vi "main.vi"() -> ()   [LabVIEW 2018]
uses:
  C:/Program Files (x86)/National Instruments/LabVIEW 2018/vi.lib/ActorFramework/Actor/Actor.lvclass
  <vilib>/ActorFramework/Message Enqueuer/Message Enqueuer.lvclass/Message Enqueuer.ctl
  <vilib>/Utility/miscctls.llb/LVPoint32TypeDef.ctl
  <vilib>/ActorFramework/Message Enqueuer/Enqueue.vi
  C:/Program Files (x86)/National Instruments/LabVIEW 2018/vi.lib/ActorFramework/Message/Message.lvclass
  <vilib>/ActorFramework/Stop Msg/Stop Msg.lvclass
  <vilib>/ActorFramework/Message Priority Queue/Priority Enqueue.vi
  <vilib>/Utility/cursorutil.llb/Set Cursor (Icon Pict).vi
  <vilib>/ActorFramework/Actor/Actor.lvclass
panel:
  out "编译执行状态":string caption="文本程序"
  in  "工具-执行":bool
  in  "工具-编译":bool
  in  "工具-导出py":bool
  in  "工具-另存为":bool
  in  "工具-保存":bool
  in  "工具-新建":bool
  in  "工具-打开":bool
  in  "工具-下载":bool
  out "保存状态":string
  out "文本程序":string
  in  "图形程序":picture[][](array[picture])
  out "备注":string[][](array[string])
  in  "辅助线":picture
  in  "连接线":picture
  in  "交互信息":string[][](array[string])
  in  "编辑控件类型":bool
  out "编辑控件":bool
  in  "全部控件":T1(array[cluster])
  in  "控件类型":cluster{"二维图片":picture, "类型名称":string}[](array[cluster])
  in  "控件列表":T2(array[cluster])
  in  "工具-帮助":bool
  in  "关键字":string[][](array[string])
  in  "执行语句":string[][](array[string])
  in  "图片名称":string[][](array[string])
  in  "停止":bool
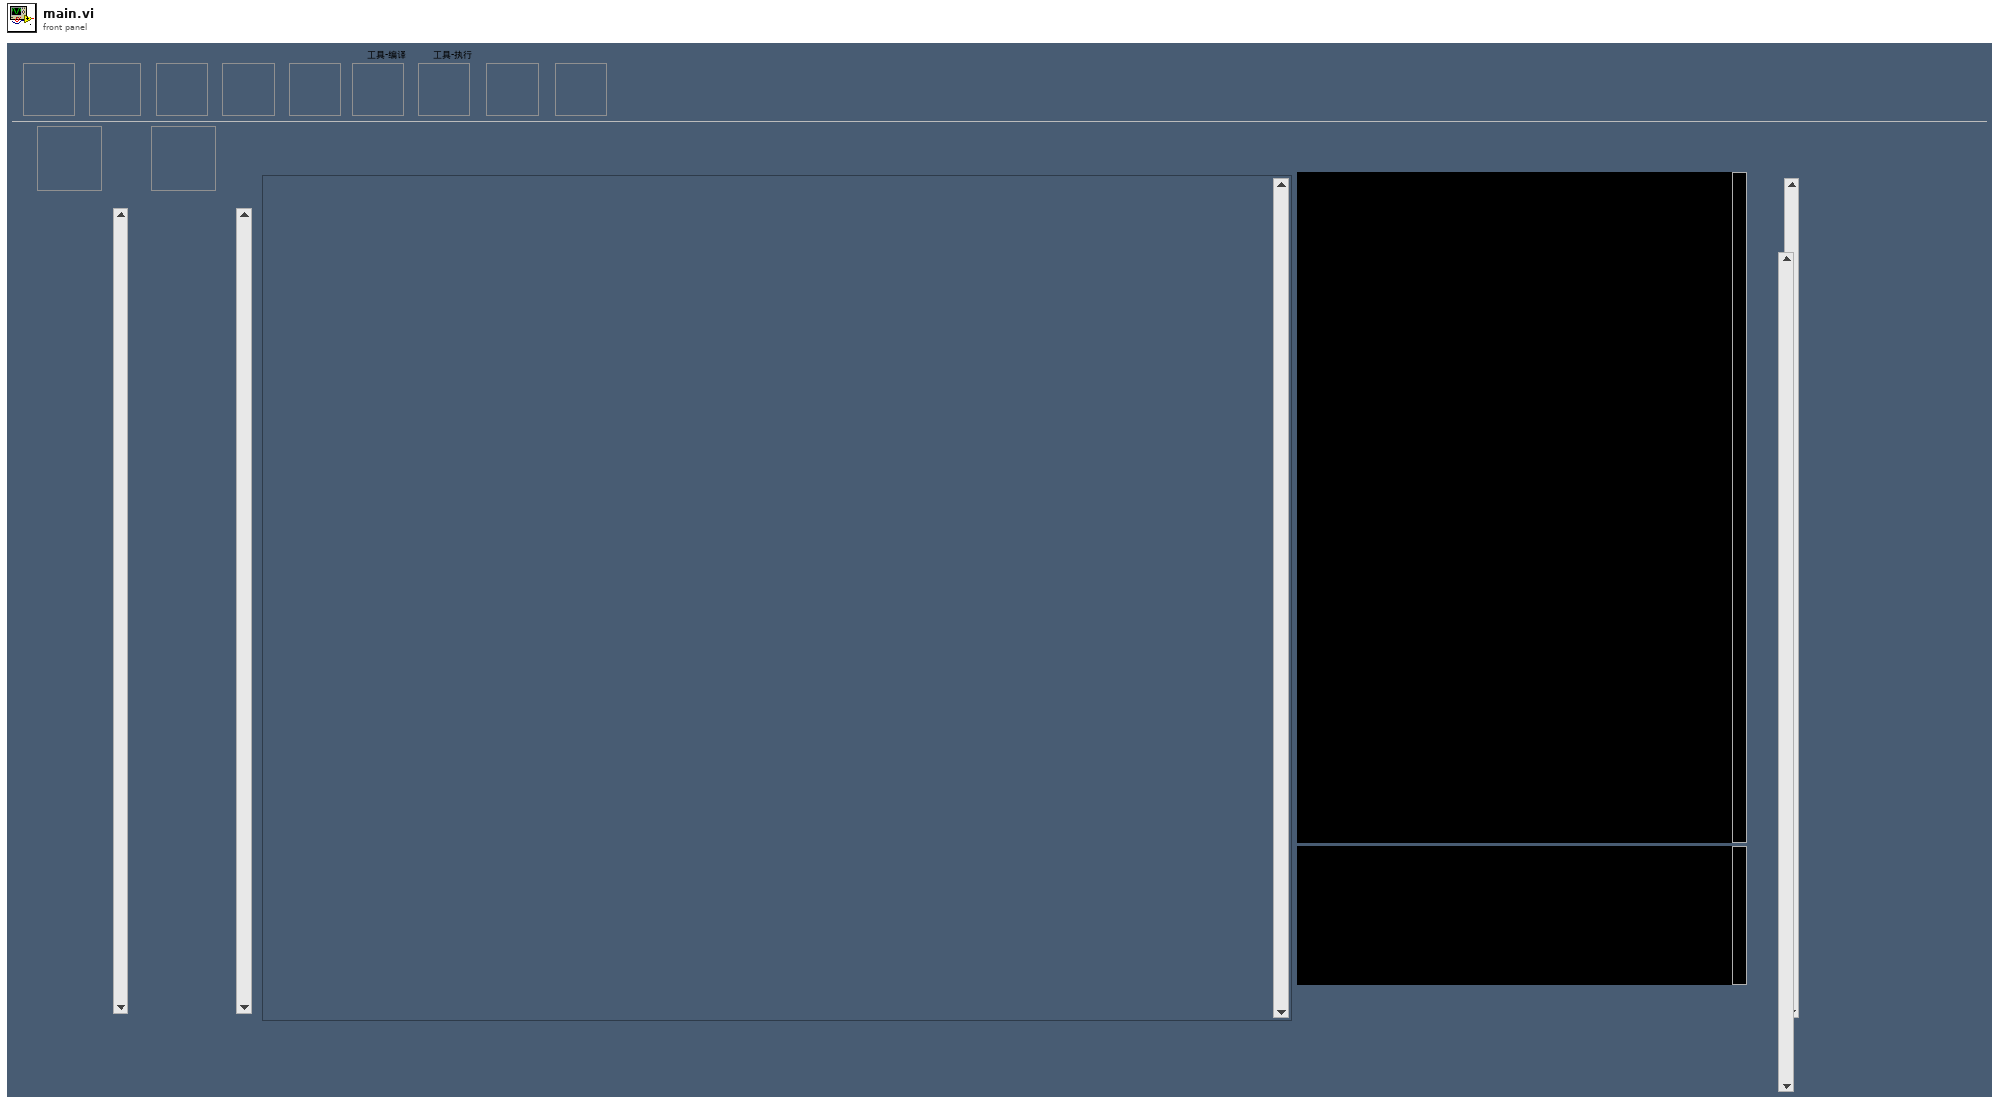
[diagram p1: front panel]
types:
  T1 = cluster{"图片":picture, "名称":string, "文本程序":string, "关键字":string}[][]
  T2 = cluster{"图片":picture, "名称":string, "文本程序":string, "关键字":string}[]
  T3 = cluster{"图形程序":refnum<vi>, "辅助线":refnum<vi>, "图片名称":refnum<vi>, "执行语句":refnum<vi>, "文本程序":refnum<vi>, "控件类型":refnum<vi>, "控件列表":refnum<vi>, "全部控件":refnum<vi>, "关键字":refnum<vi>, "连接线":refnum<vi>, "交互信息":refnum<vi>, "备注":refnum<vi>, "保存状态":refnum<vi>, "VI引用句柄":refnum<vi>, "编译执行状态":refnum<vi>}
  T4 = typedef "LVPoint32TypeDef.ctl" = cluster{"Horizontal":i32, "Vertical":i32}
  T5 = typedef "LVRectTypeDef.ctl" = cluster{"Left":i16, "Top":i16, "Right":i16, "Bottom":i16}
  T6 = typedef "LVPositionTypeDef.ctl" = cluster{"Left":i32, "Top":i32}
  T7 = typedef "eventvkey.ctl" = enum16{"ASCII", "Enter", "Return", "Shift", "Ctrl", "Alt", "Cmd", "Opt", "Caps", "NumLock", "Clear", "Break", "Up", "Down", "Left", "Right", "Insert", "Delete", "Home", "End", "PageUp", "PageDown", "Escape", "Help", "Pause", "ScrollLock", "F1", "F2", "F3", "F4", "F5", "F6", "F7", "F8", "F9", "F10", "F11", "F12", "F13", "F14", "F15", "F16", "F17", "F18", "F19", "F20", "F21", "F22", "F23", "F24", "Play", "VolumeUp", "VolumeDown", "Mute", "Two Byte Char"}
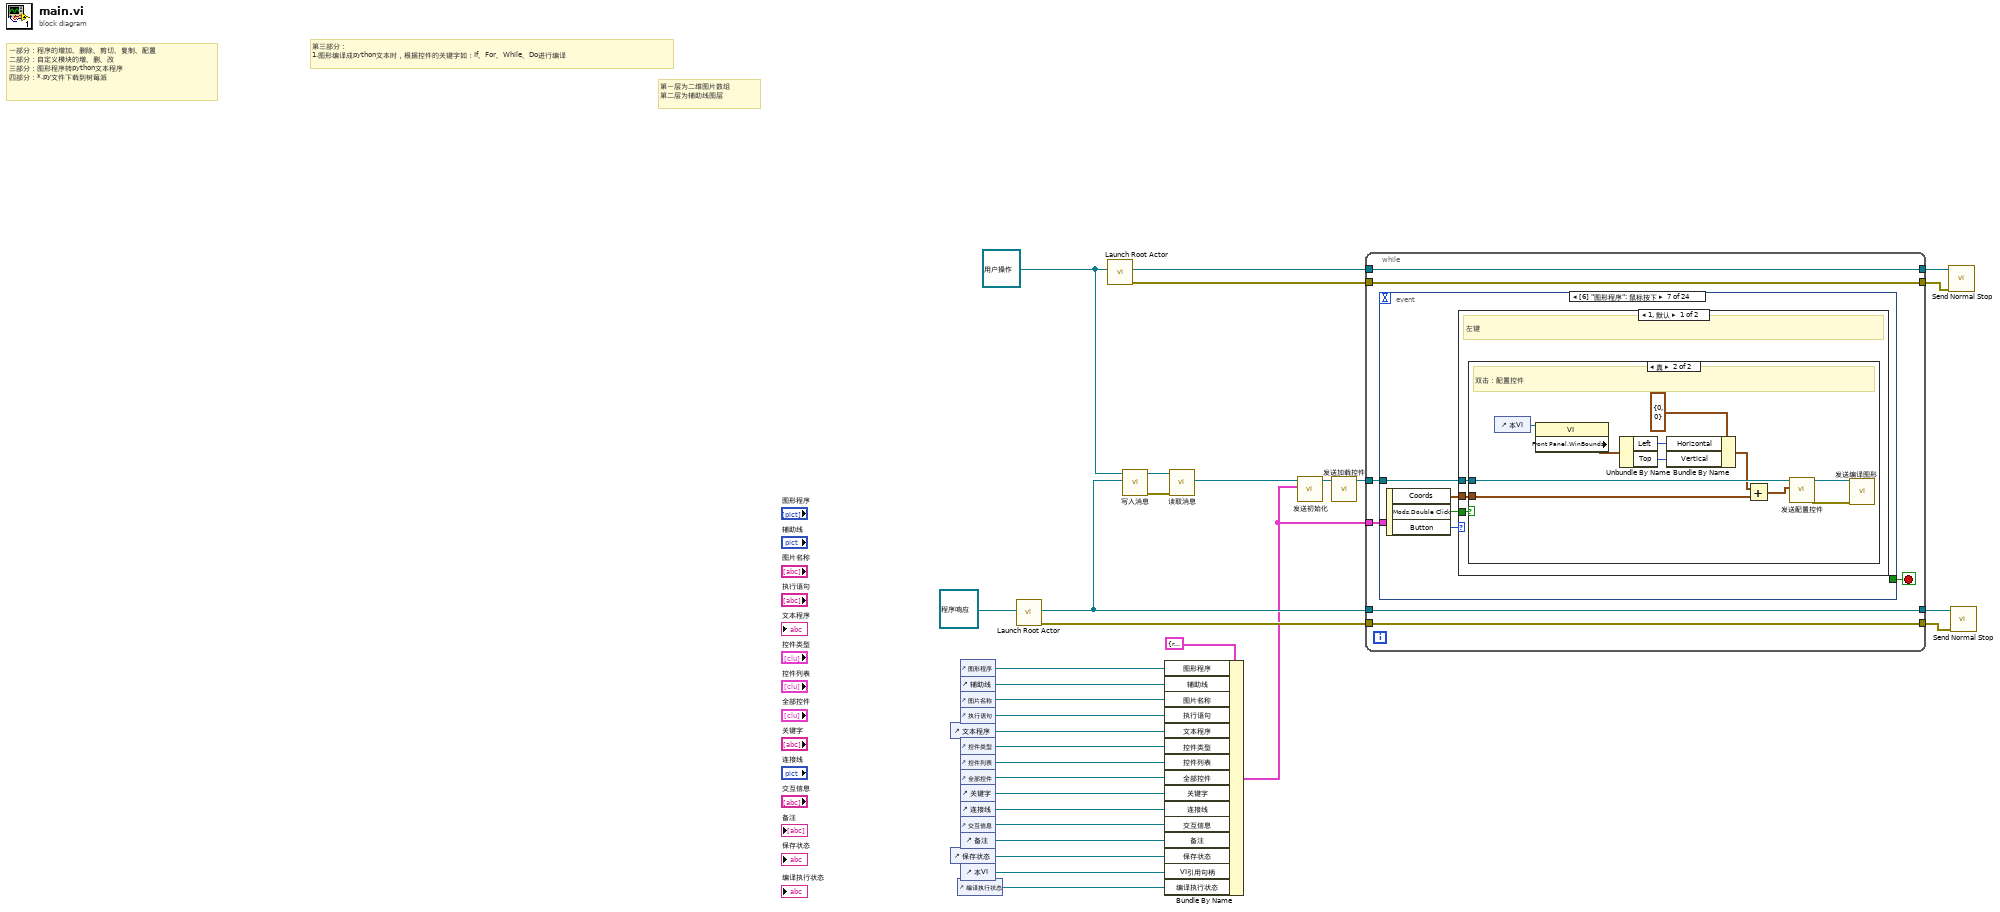
[diagram p0: block diagram]
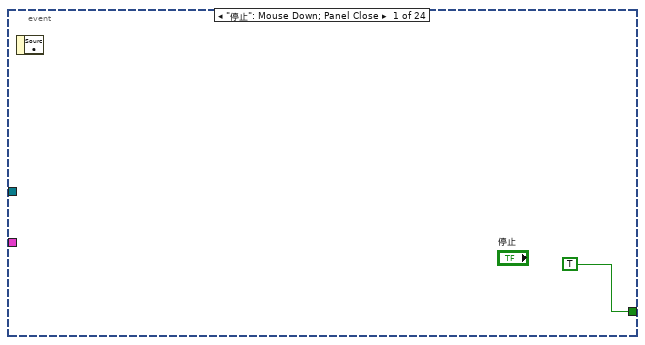
[diagram p2: hidden frame]
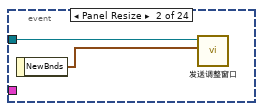
[diagram p3: hidden frame]
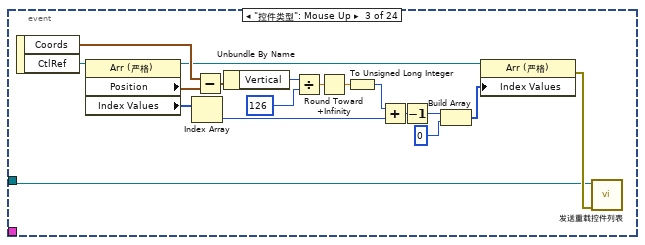
[diagram p4: hidden frame]
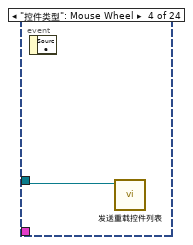
[diagram p5: hidden frame]
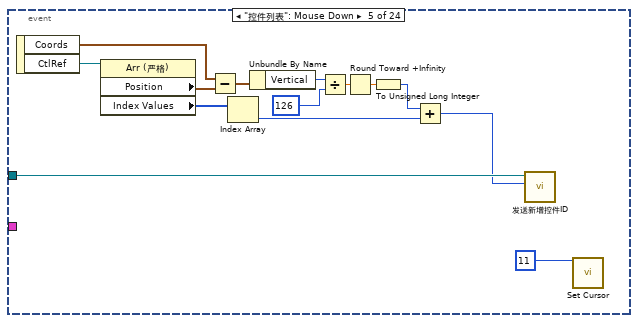
[diagram p6: hidden frame]
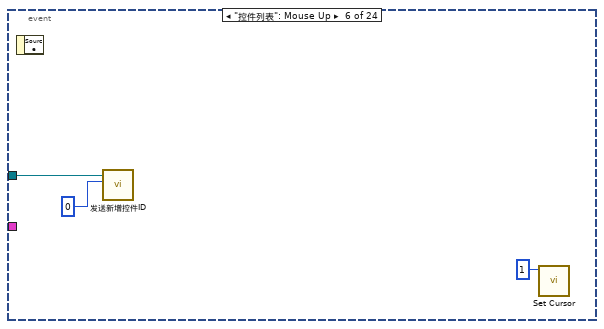
[diagram p7: hidden frame]
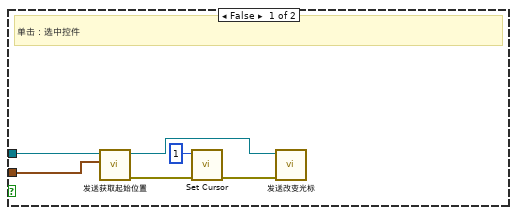
[diagram p8: hidden frame]
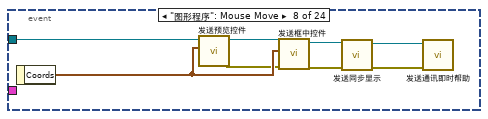
[diagram p10: hidden frame]
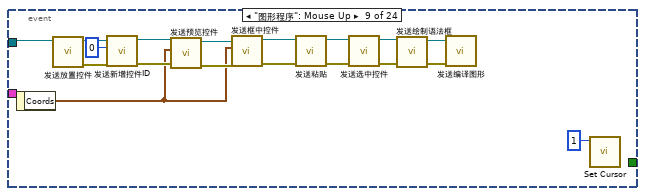
[diagram p11: hidden frame]
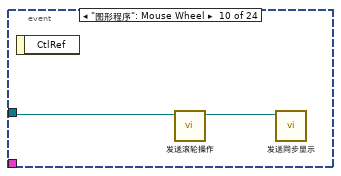
[diagram p12: hidden frame]
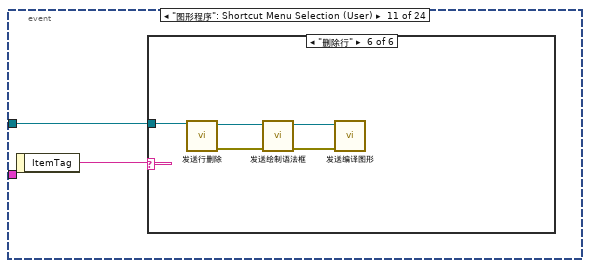
[diagram p13: hidden frame]
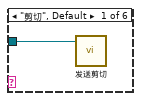
[diagram p14: hidden frame]
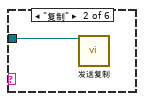
[diagram p15: hidden frame]
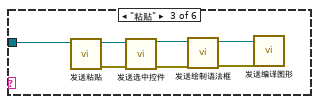
[diagram p16: hidden frame]
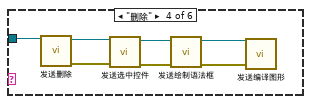
[diagram p17: hidden frame]
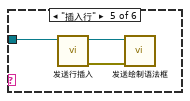
[diagram p18: hidden frame]
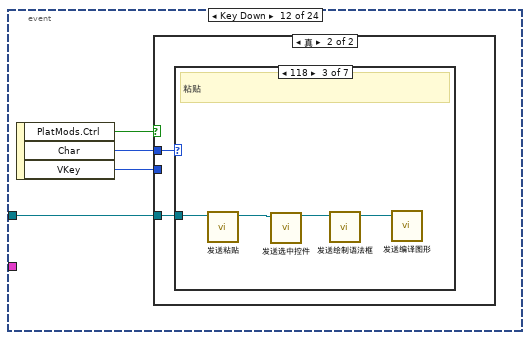
[diagram p19: hidden frame]
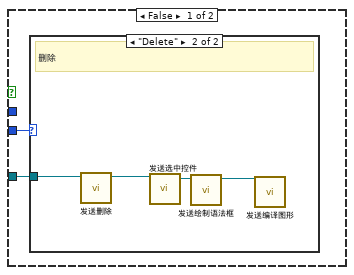
[diagram p20: hidden frame]
diagram:
  w29 = refnum<class "用户操作.lvclass"> refnum ("用户操作.lvlib:用户操作.lvclass")
  # "第三部分：\n1.图形编译成python文本时，根据控件的关键字如：If、For、While、Do进行编译"
  # "一部分：程序的增加、删除、剪切、复制、配置\n二部分：自定义模块的增、删、改\n三部分：图形程序转python文本程序\n四部分：*.py文件下载到树莓派"
  # "第一层为二维图片数组\n第二层为辅助线图层"
  n1 = control-ref of="文本程序"() -> (w16:refnum<vi>)
  n2 = control-ref of="保存状态"() -> (w7:refnum<vi>)
  n3 = control-ref of="编译执行状态"() -> (w2:refnum<vi>)
  n4 = control-ref of="图形程序"() -> (w20:refnum<vi>)
  n5 = control-ref of="辅助线"() -> (w19:refnum<vi>)
  n6 = control-ref of="图片名称"() -> (w18:refnum<vi>)
  n7 = control-ref of="执行语句"() -> (w17:refnum<vi>)
  n8 = control-ref of="控件类型"() -> (w11:refnum<vi>)
  n9 = control-ref of="控件列表"() -> (w12:refnum<vi>)
  n10 = control-ref of="全部控件"() -> (w10:refnum<vi>)
  n11 = control-ref of="关键字"() -> (w15:refnum<vi>)
  n12 = control-ref of="连接线"() -> (w14:refnum<vi>)
  n13 = control-ref of="交互信息"() -> (w9:refnum<vi>)
  n14 = control-ref of="备注"() -> (w8:refnum<vi>)
  n15 = control-ref of="本VI"() -> (w5:refnum<vi>)
  n16 = call <vilib>:"Launch Root Actor.vi"("Actor"=refnum<class "程序响应.lvclass"> refnum ("程序响应.lvlib:程序响应.lvclass")) -> ("error out"=w24:errorcluster, "Actor's Enqueuer"=w28:refnum<class "Message Enqueuer.lvclass">)  [unwired: 9 in]
  n17 = call <vilib>:"Launch Root Actor.vi"("Actor"=w29) -> ("error out"=w22:errorcluster, "Actor's Enqueuer"=w27:refnum<class "Message Enqueuer.lvclass">)  [unwired: 9 in]
  n18 = call-dynamic "写入消息.vi"("操作者框架:消息待入队列"=w28, "用户操作输入"=w29) -> ("error out"=w30:errorcluster, "用户操作输出"=w31:refnum<class "用户操作.lvclass">)  [unwired: 8 in]
  n19 = Bundle By Name(cluster=T3 {"图形程序"=refnum, "辅助线"=refnum, "图片名称"=refnum, "执行语句"=refnum, "文本程序"=refnum, "控件类型"=refnum, "控件列表"=refnum, "全部控件"=refnum, "关键字"=refnum, "连接线"=refnum, "交互信息"=refnum, "备注"=refnum, "保存状态"=refnum, "VI引用句柄"=refnum, "编译执行状态"=refnum} ("初始数据"), "图形程序"=w20, "辅助线"=w19, "图片名称"=w18, "执行语句"=w17, "文本程序"=w16, "控件类型"=w11, "控件列表"=w12, "全部控件"=w10, "关键字"=w15, "连接线"=w14, "交互信息"=w9, "备注"=w8, "保存状态"=w7, "VI引用句柄"=w5, "编译执行状态"=w2) -> (w1:T3)
  n20 = call-dynamic "读取消息.vi"("error in (no error)"=w30, "用户操作输入"=w31) -> ("操作者框架:消息待入队列"=w4:refnum<class "Message Enqueuer.lvclass">)  [unwired: 7 in, 2 out]
  n21 = call "发送初始化.vi"("初始数据"=w1, "Message Enqueuer"=w4) -> ("Message Enqueuer out"=w3:refnum<class "Message Enqueuer.lvclass">)  [unwired: 8 in, 1 out]
  n22 = call "发送加载控件.vi"("Message Enqueuer"=w3) -> ("Message Enqueuer out"=w13:refnum<class "Message Enqueuer.lvclass">)  [unwired: 9 in, 1 out]
  n23 = while {
    tunnel: w28 -> [w37]
    tunnel: w13 -> [w39]
    tunnel: w27 -> [w38]
    tunnel: [w38] -> w26
    tunnel: [w37] -> w25
    tunnel: w24 -> [w36]
    tunnel: [w36] -> w23
    tunnel: w22 -> [w35]
    tunnel: [w35] -> w21
    tunnel: w1 -> [w33]
    stop <- w34 stop-if-true
    n24 = event shown="[6] \"图形程序\": 鼠标按下" {
      selector: _ -> [_ _ _ _ _ _ _ _ _ _ _ _ _ _ _ _ _ _ _ _ _ _ _ _]
      dyn-events: _ -> [_ _ _ _ _ _ _ _ _ _ _ _ _ _ _ _ _ _ _ _ _ _ _ _]
      timeout: _ -> [_ _ _ _ _ _ _ _ _ _ _ _ _ _ _ _ _ _ _ _ _ _ _ _]
      tunnel: w39 -> [_ w42 w43 w61 w66 w78 w82 w110 w125 w129 w131 w157 w183 w186 w188 w193 w194 w195 w197 w198 w199 w201 w202 w204]
      tunnel: [TRUE _ _ _ _ _ _ _ _ _ _ _ _ _ _ _ _ _ _ _ _ _ _ _] -> w34
      tunnel: w33 -> [_ _ _ _ _ _ _ _ _ _ _ _ _ _ w187 _ _ _ _ _ _ _ _ _]
      event "停止": Mouse Down; Panel Close {
        n25 = event-data() -> ()  [unwired: 1 in, 1 out]
      }
      event Panel Resize {
        n26 = event-data() -> ("NewBnds"=w41:T5)  [unwired: 1 in]
        n27 = call "发送调整窗口.vi"("前面板范围"=w41, "Message Enqueuer"=w42) -> ()  [unwired: 8 in, 2 out]
      }
      event "控件类型": Mouse Up {
        n28 = event-data() -> ("Coords"=w51:T4, "CtlRef"=w50:refnum<vi>)  [unwired: 1 in]
        n29 = property class="Arr (严格)"(reference=w50) -> (reference out=w49:refnum<vi>, "Position"=w60:T6, "Index Values"=w55:u32[])  [unwired: 1 in, 1 out]
        n30 = Index Array(array=w55) -> (element=w54:u32)  [unwired: 1 in]
        n31 = Subtract(x=w51, y=w60) -> (x-y=w59:T4)
        n32 = Unbundle By Name(w59) -> ("Vertical"=w58:i32)
        n33 = Divide(x=w58, y=126) -> (x/y=w56:dbl)
        n34 = Round Toward +Infinity(x=w56) -> (ceil(x): smallest int >= x=w53:dbl)
        n35 = To Unsigned Long Integer(number=w53) -> (unsigned 32bit integer=w52:u32)
        n36 = Add(x=w52, y=w54) -> (x+y=w48:u32)
        n37 = Decrement(x=w48) -> (x-1=w45:u32)
        n38 = Build Array(w45, u32 0 ("元素")) -> (w46:u32[])
        n39 = property class="Arr (严格)"(reference=w49, "Index Values"=w46) -> (error out=w44:errorcluster)  [unwired: 1 in, 1 out]
        n40 = call "发送重载控件列表.vi"("error in (no error)"=w44, "Message Enqueuer"=w43) -> ()  [unwired: 8 in, 2 out]
      }
      event "控件类型": Mouse Wheel {
        n41 = event-data() -> ()  [unwired: 1 in, 1 out]
        n42 = call "发送重载控件列表.vi"("Message Enqueuer"=w61) -> ()  [unwired: 9 in, 2 out]
      }
      event "控件列表": Mouse Down {
        n43 = event-data() -> ("Coords"=w62:T4, "CtlRef"=w64:refnum<vi>)  [unwired: 1 in]
        n44 = property class="Arr (严格)"(reference=w64) -> ("Position"=w75:T6, "Index Values"=w70:u32[])  [unwired: 1 in, 2 out]
        n45 = Subtract(x=w62, y=w75) -> (x-y=w74:T4)
        n46 = Index Array(array=w70) -> (element=w69:u32)  [unwired: 1 in]
        n47 = Unbundle By Name(w74) -> ("Vertical"=w73:i32)
        n48 = Divide(x=w73, y=126) -> (x/y=w71:dbl)
        n49 = Round Toward +Infinity(x=w71) -> (ceil(x): smallest int >= x=w68:dbl)
        n50 = To Unsigned Long Integer(number=w68) -> (unsigned 32bit integer=w67:u32)
        n51 = Add(x=w67, y=w69) -> (x+y=w63:u32)
        n52 = call "发送新增控件ID.vi"("控件ID"=w63, "Message Enqueuer"=w66) -> ()  [unwired: 8 in, 2 out]
        n53 = call-poly <vilib>:"Set Cursor.vi"("icon"=u16 11) -> ()  [unwired: 9 in, 2 out]
      }
      event "控件列表": Mouse Up {
        n54 = event-data() -> ()  [unwired: 1 in, 1 out]
        n55 = call "发送新增控件ID.vi"("控件ID"=u32 0, "Message Enqueuer"=w78) -> ()  [unwired: 8 in, 2 out]
        n56 = call-poly <vilib>:"Set Cursor.vi"("icon"=u16 1) -> ()  [unwired: 9 in, 2 out]
      }
      event "图形程序": Mouse Down {
        n57 = event-data() -> ("Coords"=w81:T4, "Mods.Double Click"=w79:bool, "Button"=w80:u16)  [unwired: 1 in]
        n58 = case shown="1, 默认" w80 {
          tunnel: w82 -> [w85 _]
          tunnel: w81 -> [w84 _]
          tunnel: w79 -> [w83 _]
          frame 1, Default {
            # "左键"
            n59 = case shown="真" w83 {
              tunnel: w85 -> [w91 w102]
              tunnel: w84 -> [w90 w100]
              frame False {
                # "单击：选中控件"
                n60 = call "发送获取起始位置.vi"("起始坐标"=w90, "Message Enqueuer"=w91) -> ("error out"=w88:errorcluster, "Message Enqueuer out"=w86:refnum<class "Message Enqueuer.lvclass">)  [unwired: 8 in]
                n61 = call-poly <vilib>:"Set Cursor.vi"("error in (no error)"=w88, "icon"=u16 1) -> ("error out"=w87:errorcluster)  [unwired: 8 in, 1 out]
                n62 = call "发送改变光标.vi"("error in (no error)"=w87, "Message Enqueuer"=w86) -> ()  [unwired: 8 in, 2 out]
              }
              frame True {
                # "双击：配置控件"
                n63 = control-ref of="本VI"() -> (w101:refnum<vi>)
                n64 = property class="VI"(reference=w101) -> ("Front Panel.WinBounds"=w98:T5)  [unwired: 1 in, 2 out]
                n65 = Unbundle By Name(w98) -> ("Left"=w97:i16, "Top"=w96:i16)
                n66 = Bundle By Name(cluster=T4 {"Horizontal"=0, "Vertical"=0} ("x"), "Horizontal"=w97, "Vertical"=w96) -> (w94:T4)
                n67 = Add(x=w94, y=w100) -> (x+y=w99:T4)
                n68 = call "发送配置控件.vi"("鼠标位置"=w99, "Message Enqueuer"=w102) -> ("error out"=w92:errorcluster, "Message Enqueuer out"=w93:refnum<class "Message Enqueuer.lvclass">)  [unwired: 8 in]
                n69 = call "发送编译图形.vi"("error in (no error)"=w92, "Message Enqueuer"=w93) -> ()  [unwired: 8 in, 2 out]
              }
            }
          }
          frame 2 {
            # "右键自定义菜单"
          }
        }
      }
      event "图形程序": Mouse Move {
        n70 = event-data() -> ("Coords"=w108:T4)  [unwired: 1 in]
        n71 = call "发送预览控件.vi"("鼠标位置"=w108, "Message Enqueuer"=w110) -> ("error out"=w107:errorcluster, "Message Enqueuer out"=w109:refnum<class "Message Enqueuer.lvclass">)  [unwired: 8 in]
        n72 = call "发送框中控件.vi"("error in (no error)"=w107, "结束坐标"=w108, "Message Enqueuer"=w109) -> ("error out"=w105:errorcluster, "Message Enqueuer out"=w106:refnum<class "Message Enqueuer.lvclass">)  [unwired: 7 in]
        n73 = call "发送同步显示.vi"("error in (no error)"=w105, "Message Enqueuer"=w106) -> ("error out"=w103:errorcluster, "Message Enqueuer out"=w104:refnum<class "Message Enqueuer.lvclass">)  [unwired: 8 in]
        n74 = call "发送通讯即时帮助.vi"("error in (no error)"=w103, "Message Enqueuer"=w104) -> ()  [unwired: 8 in, 2 out]
      }
      event "图形程序": Mouse Up {
        n75 = event-data() -> ("Coords"=w120:T4)  [unwired: 1 in]
        n76 = call "发送放置控件.vi"("Message Enqueuer"=w125) -> ("error out"=w126:errorcluster, "Message Enqueuer out"=w127:refnum<class "Message Enqueuer.lvclass">)  [unwired: 9 in]
        n77 = call "发送新增控件ID.vi"("error in (no error)"=w126, "控件ID"=u32 0, "Message Enqueuer"=w127) -> ("error out"=w123:errorcluster, "Message Enqueuer out"=w124:refnum<class "Message Enqueuer.lvclass">)  [unwired: 7 in]
        n78 = call "发送预览控件.vi"("error in (no error)"=w123, "鼠标位置"=w120, "Message Enqueuer"=w124) -> ("error out"=w121:errorcluster, "Message Enqueuer out"=w122:refnum<class "Message Enqueuer.lvclass">)  [unwired: 7 in]
        n79 = call "发送框中控件.vi"("error in (no error)"=w121, "结束坐标"=w120, "Message Enqueuer"=w122) -> ("error out"=w113:errorcluster, "Message Enqueuer out"=w114:refnum<class "Message Enqueuer.lvclass">)  [unwired: 7 in]
        n80 = call "发送粘贴.vi"("error in (no error)"=w113, "Message Enqueuer"=w114) -> ("error out"=w111:errorcluster, "Message Enqueuer out"=w112:refnum<class "Message Enqueuer.lvclass">)  [unwired: 8 in]
        n81 = call "发送选中控件.vi"("error in (no error)"=w111, "Message Enqueuer"=w112) -> ("error out"=w115:errorcluster, "Message Enqueuer out"=w116:refnum<class "Message Enqueuer.lvclass">)  [unwired: 8 in]
        n82 = call "发送绘制语法框.vi"("error in (no error)"=w115, "Message Enqueuer"=w116) -> ("error out"=w117:errorcluster, "Message Enqueuer out"=w118:refnum<class "Message Enqueuer.lvclass">)  [unwired: 8 in]
        n83 = call "发送编译图形.vi"("error in (no error)"=w117, "Message Enqueuer"=w118) -> ()  [unwired: 8 in, 2 out]
        n84 = call-poly <vilib>:"Set Cursor.vi"("icon"=u16 1) -> ()  [unwired: 9 in, 2 out]
      }
      event "图形程序": Mouse Wheel {
        n85 = event-data() -> ()  [unwired: 1 in, 1 out]
        n86 = call "发送滚轮操作.vi"("Message Enqueuer"=w129) -> ("Message Enqueuer out"=w130:refnum<class "Message Enqueuer.lvclass">)  [unwired: 9 in, 1 out]
        n87 = call "发送同步显示.vi"("Message Enqueuer"=w130) -> ()  [unwired: 9 in, 2 out]
      }
      event "图形程序": Shortcut Menu Selection (User) {
        n88 = event-data() -> ("ItemTag"=w132:string)  [unwired: 1 in]
        n89 = case shown="\"删除行\"" w132 {
          tunnel: w131 -> [w133 w134 w141 w148 w151 w156]
          frame "剪切", Default {
            n90 = call "发送剪切.vi"("Message Enqueuer"=w133) -> ()  [unwired: 9 in, 2 out]
          }
          frame "复制" {
            n91 = call "发送复制.vi"("Message Enqueuer"=w134) -> ()  [unwired: 9 in, 2 out]
          }
          frame "粘贴" {
            n92 = call "发送粘贴.vi"("Message Enqueuer"=w141) -> ("error out"=w137:errorcluster, "Message Enqueuer out"=w140:refnum<class "Message Enqueuer.lvclass">)  [unwired: 9 in]
            n93 = call "发送选中控件.vi"("error in (no error)"=w137, "Message Enqueuer"=w140) -> ("error out"=w136:errorcluster, "Message Enqueuer out"=w139:refnum<class "Message Enqueuer.lvclass">)  [unwired: 8 in]
            n94 = call "发送绘制语法框.vi"("error in (no error)"=w136, "Message Enqueuer"=w139) -> ("error out"=w135:errorcluster, "Message Enqueuer out"=w138:refnum<class "Message Enqueuer.lvclass">)  [unwired: 8 in]
            n95 = call "发送编译图形.vi"("error in (no error)"=w135, "Message Enqueuer"=w138) -> ()  [unwired: 8 in, 2 out]
          }
          frame "删除" {
            n96 = call "发送删除.vi"("Message Enqueuer"=w148) -> ("error out"=w144:errorcluster, "Message Enqueuer out"=w147:refnum<class "Message Enqueuer.lvclass">)  [unwired: 9 in]
            n97 = call "发送选中控件.vi"("error in (no error)"=w144, "Message Enqueuer"=w147) -> ("error out"=w143:errorcluster, "Message Enqueuer out"=w146:refnum<class "Message Enqueuer.lvclass">)  [unwired: 8 in]
            n98 = call "发送绘制语法框.vi"("error in (no error)"=w143, "Message Enqueuer"=w146) -> ("error out"=w142:errorcluster, "Message Enqueuer out"=w145:refnum<class "Message Enqueuer.lvclass">)  [unwired: 8 in]
            n99 = call "发送编译图形.vi"("error in (no error)"=w142, "Message Enqueuer"=w145) -> ()  [unwired: 8 in, 2 out]
          }
          frame "插入行" {
            n100 = call "发送行插入.vi"("Message Enqueuer"=w151) -> ("error out"=w149:errorcluster, "Message Enqueuer out"=w150:refnum<class "Message Enqueuer.lvclass">)  [unwired: 9 in]
            n101 = call "发送绘制语法框.vi"("error in (no error)"=w149, "Message Enqueuer"=w150) -> ()  [unwired: 8 in, 2 out]
          }
          frame "删除行" {
            n102 = call "发送行删除.vi"("Message Enqueuer"=w156) -> ("error out"=w153:errorcluster, "Message Enqueuer out"=w155:refnum<class "Message Enqueuer.lvclass">)  [unwired: 9 in]
            n103 = call "发送绘制语法框.vi"("error in (no error)"=w153, "Message Enqueuer"=w155) -> ("error out"=w152:errorcluster, "Message Enqueuer out"=w154:refnum<class "Message Enqueuer.lvclass">)  [unwired: 8 in]
            n104 = call "发送编译图形.vi"("error in (no error)"=w152, "Message Enqueuer"=w154) -> ()  [unwired: 8 in, 2 out]
          }
        }
      }
      event Key Down {
        n105 = event-data() -> ("PlatMods.Ctrl"=w160:bool, "Char"=w159:i16, "VKey"=w158:T7)  [unwired: 1 in]
        n106 = case shown="真" w160 {
          tunnel: w159 -> [_ w168]
          tunnel: w158 -> [w162 _]
          tunnel: w157 -> [w161 w167]
          frame False {
            n107 = case shown="\"Delete\"" w162 {
              tunnel: w161 -> [_ w165]
              frame "ASCII", Default {
              }
              frame "Delete" {
                # "删除"
                n108 = call "发送删除.vi"("Message Enqueuer"=w165) -> ("Message Enqueuer out"=w166:refnum<class "Message Enqueuer.lvclass">)  [unwired: 9 in, 1 out]
                n109 = call "发送选中控件.vi"("Message Enqueuer"=w166) -> ("Message Enqueuer out"=w164:refnum<class "Message Enqueuer.lvclass">)  [unwired: 9 in, 1 out]
                n110 = call "发送绘制语法框.vi"("Message Enqueuer"=w164) -> ("Message Enqueuer out"=w163:refnum<class "Message Enqueuer.lvclass">)  [unwired: 9 in, 1 out]
                n111 = call "发送编译图形.vi"("Message Enqueuer"=w163) -> ()  [unwired: 9 in, 2 out]
              }
            }
          }
          frame True {
            n112 = case shown="118" w168 {
              tunnel: w167 -> [_ w169 w173 w174 w175 w178 w180]
              frame 0, Default {
              }
              frame 99 {
                # "复制"
                n113 = call "发送复制.vi"("Message Enqueuer"=w169) -> ()  [unwired: 9 in, 2 out]
              }
              frame 118 {
                # "粘贴"
                n114 = call "发送粘贴.vi"("Message Enqueuer"=w173) -> ("Message Enqueuer out"=w172:refnum<class "Message Enqueuer.lvclass">)  [unwired: 9 in, 1 out]
                n115 = call "发送选中控件.vi"("Message Enqueuer"=w172) -> ("Message Enqueuer out"=w171:refnum<class "Message Enqueuer.lvclass">)  [unwired: 9 in, 1 out]
                n116 = call "发送绘制语法框.vi"("Message Enqueuer"=w171) -> ("Message Enqueuer out"=w170:refnum<class "Message Enqueuer.lvclass">)  [unwired: 9 in, 1 out]
                n117 = call "发送编译图形.vi"("Message Enqueuer"=w170) -> ()  [unwired: 9 in, 2 out]
              }
              frame 120 {
                # "剪切"
                n118 = call "发送剪切.vi"("Message Enqueuer"=w174) -> ()  [unwired: 9 in, 2 out]
              }
              frame 97 {
                # "CTRL+A插入行"
                n119 = call "发送行插入.vi"("Message Enqueuer"=w175) -> ("Message Enqueuer out"=w176:refnum<class "Message Enqueuer.lvclass">)  [unwired: 9 in, 1 out]
                n120 = call "发送绘制语法框.vi"("Message Enqueuer"=w176) -> ()  [unwired: 9 in, 2 out]
              }
              frame 100 {
                # "CTRL+D删除行"
                n121 = call "发送行删除.vi"("Message Enqueuer"=w178) -> ("Message Enqueuer out"=w179:refnum<class "Message Enqueuer.lvclass">)  [unwired: 9 in, 1 out]
                n122 = call "发送绘制语法框.vi"("Message Enqueuer"=w179) -> ("Message Enqueuer out"=w177:refnum<class "Message Enqueuer.lvclass">)  [unwired: 9 in, 1 out]
                n123 = call "发送编译图形.vi"("Message Enqueuer"=w177) -> ()  [unwired: 9 in, 2 out]
              }
              frame 115 {
                # "保存文件"
                n124 = call "发送菜单-保存.vi"("Message Enqueuer"=w180) -> ()  [unwired: 9 in, 2 out]
              }
            }
          }
        }
      }
      event "编辑控件类型": Mouse Up {
        n125 = event-data() -> ()  [unwired: 1 in, 1 out]
        n126 = call "发送编辑控件类型.vi"("Message Enqueuer"=w183) -> ("error out"=w181:errorcluster, "Message Enqueuer out"=w182:refnum<class "Message Enqueuer.lvclass">)  [unwired: 9 in]
        n127 = call "发送加载控件.vi"("error in (no error)"=w181, "Message Enqueuer"=w182) -> ()  [unwired: 8 in, 2 out]
      }
      event "编辑控件": Mouse Up {
        n128 = event-data() -> ()  [unwired: 1 in, 1 out]
        n129 = call "发送编辑控件.vi"("Message Enqueuer"=w186) -> ("error out"=w184:errorcluster, "Message Enqueuer out"=w185:refnum<class "Message Enqueuer.lvclass">)  [unwired: 9 in]
        n130 = call "发送加载控件.vi"("error in (no error)"=w184, "Message Enqueuer"=w185) -> ()  [unwired: 8 in, 2 out]
      }
      event "工具-新建": Mouse Up {
        n131 = event-data() -> ()  [unwired: 1 in, 1 out]
        n132 = call "发送初始化.vi"("初始数据"=w187, "Message Enqueuer"=w188) -> ()  [unwired: 8 in, 2 out]
      }
      event "工具-打开": Mouse Up {
        n133 = event-data() -> ()  [unwired: 1 in, 1 out]
        n134 = call "发送菜单-打开.vi"("Message Enqueuer"=w193) -> ("error out"=w189:errorcluster, "Message Enqueuer out"=w192:refnum<class "Message Enqueuer.lvclass">)  [unwired: 9 in]
        n135 = call "发送绘制语法框.vi"("error in (no error)"=w189, "Message Enqueuer"=w192) -> ("error out"=w190:errorcluster, "Message Enqueuer out"=w191:refnum<class "Message Enqueuer.lvclass">)  [unwired: 8 in]
        n136 = call "发送编译图形.vi"("error in (no error)"=w190, "Message Enqueuer"=w191) -> ()  [unwired: 8 in, 2 out]
      }
      event "工具-保存": Mouse Up {
        n137 = event-data() -> ()  [unwired: 1 in, 1 out]
        n138 = call "发送菜单-保存.vi"("Message Enqueuer"=w194) -> ()  [unwired: 9 in, 2 out]
      }
      event "工具-另存为": Mouse Up {
        n139 = event-data() -> ()  [unwired: 1 in, 1 out]
        n140 = call "发送菜单-另存为.vi"("Message Enqueuer"=w195) -> ()  [unwired: 9 in, 2 out]
      }
      event "工具-导出py": Mouse Up {
        n141 = event-data() -> ()  [unwired: 1 in, 1 out]
        n142 = call "发送编译图形.vi"("Message Enqueuer"=w197) -> ("Message Enqueuer out"=w196:refnum<class "Message Enqueuer.lvclass">)  [unwired: 9 in, 1 out]
        n143 = call "发送菜单-导出py.vi"("Message Enqueuer"=w196) -> ()  [unwired: 9 in, 2 out]
      }
      event "工具-编译": Mouse Up {
        n144 = event-data() -> ()  [unwired: 1 in, 1 out]
        n145 = call "发送菜单-编译.vi"("Message Enqueuer"=w198) -> ()  [unwired: 9 in, 2 out]
      }
      event "工具-执行": Mouse Up {
        n146 = event-data() -> ()  [unwired: 1 in, 1 out]
        n147 = call "发送菜单-执行.vi"("Message Enqueuer"=w199) -> ()  [unwired: 9 in, 2 out]
      }
      event "工具-下载": Mouse Up {
        n148 = event-data() -> ()  [unwired: 1 in, 1 out]
        n149 = call "发送编译图形.vi"("Message Enqueuer"=w201) -> ("Message Enqueuer out"=w200:refnum<class "Message Enqueuer.lvclass">)  [unwired: 9 in, 1 out]
        n150 = call "发送菜单-下载.vi"("Message Enqueuer"=w200) -> ()  [unwired: 9 in, 2 out]
      }
      event "工具-帮助": Mouse Up {
        n151 = event-data() -> ()  [unwired: 1 in, 1 out]
        n152 = call "发送显示帮助信息.vi"("Message Enqueuer"=w202) -> ()  [unwired: 9 in, 2 out]
      }
      event "文本程序": Mouse Down {
        n153 = event-data() -> ("Button"=w203:u16)  [unwired: 1 in]
        n154 = case shown="2" w203 {
          tunnel: w204 -> [_ w205]
          frame 0, Default {
          }
          frame 2 {
            n155 = call "发送设置字体.vi"("Message Enqueuer"=w205) -> ()  [unwired: 9 in, 2 out]
          }
        }
      }
    }
  }
  n156 = call <vilib>:"Send Normal Stop.vi"("error in (no error)"=w21, "Message Enqueuer"=w26) -> ()  [unwired: 9 in, 1 out]
  n157 = call <vilib>:"Send Normal Stop.vi"("error in (no error)"=w23, "Message Enqueuer"=w25) -> ()  [unwired: 9 in, 1 out]
